vi "Make RomiGyro JSON.vi"(9 "Force":bool, 10 "Previous":T1={"type"="AI", "device"="", "name"="", "data"={"<init"=0, ">connected"=FALSE, "<offsetX"=0.0, "<offsetY"=0.0, "<offsetZ"=0.0, ">angle_x"=0.0, ">angle_y"=0.0, ">angle_z"=0.0, ">rate_x"=0.0, ">rate_y"=0.0, ">rate_z"=0.0, "<gain"=0.0}}, 11 "New":T1={"type"="AI", "device"="", "name"="", "data"={"<init"=0, ">connected"=FALSE, "<offsetX"=0.0, "<offsetY"=0.0, "<offsetZ"=0.0, ">angle_x"=0.0, ">angle_y"=0.0, ">angle_z"=0.0, ">rate_x"=0.0, ">rate_y"=0.0, ">rate_z"=0.0, "<gain"=0.0}}) -> (3 "delta JSON":string)   [LabVIEW 2019]
uses:
  RomiGyro Data proto.ctl
  RomiGyro proto.ctl
panel:
  out "Complete JSON":string
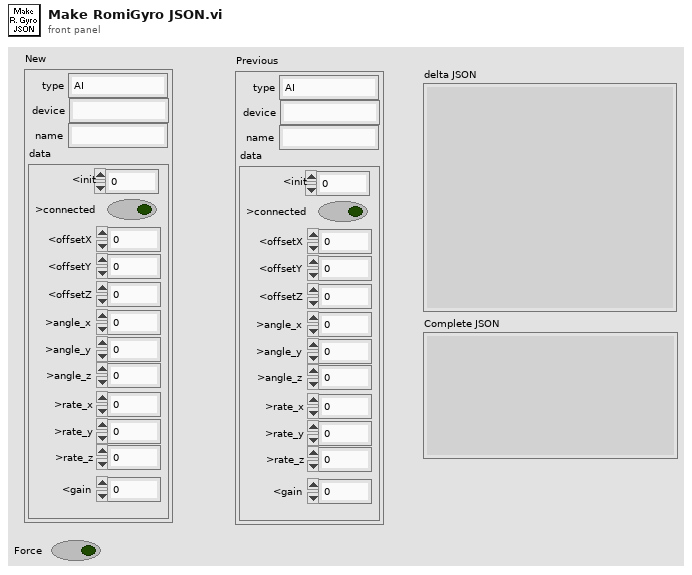
[diagram p1: front panel]
types:
  T1 = typedef "RomiGyro proto.ctl" = cluster{"type":string, "device":string, "name":string, "data":T2}
  T2 = typedef "RomiGyro Data proto.ctl" = cluster{"<init":i32, ">connected":bool, "<offsetX":dbl, "<offsetY":dbl, "<offsetZ":dbl, ">angle_x":dbl, ">angle_y":dbl, ">angle_z":dbl, ">rate_x":dbl, ">rate_y":dbl, ">rate_z":dbl, "<gain":dbl}
  T3 = cluster{"type":bool, "device":bool, "name":bool, "data":cluster{"<init":bool, ">connected":bool, "<offsetX":bool, "<offsetY":bool, "<offsetZ":bool, ">angle_x":bool, ">angle_y":bool, ">angle_z":bool, ">rate_x":bool, ">rate_y":bool, ">rate_z":bool, "<gain":bool}}
  T4 = cluster{"<init":bool, ">connected":bool, "<offsetX":bool, "<offsetY":bool, "<offsetZ":bool, ">angle_x":bool, ">angle_y":bool, ">angle_z":bool, ">rate_x":bool, ">rate_y":bool, ">rate_z":bool, "<gain":bool}
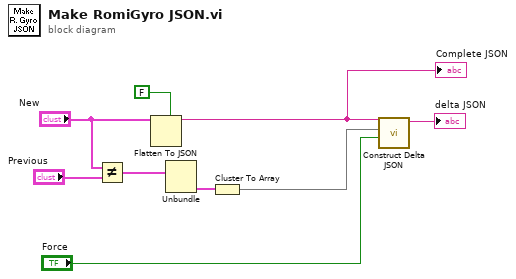
[diagram p0: block diagram]
diagram:
  n1 = Not Equal?(x="New", y="Previous") -> (x != y?=w6:T3)
  n2 = Flatten To JSON(enable LabVIEW extensions? (T)=FALSE, anything="New") -> (JSON string=w5:string)  [unwired: 1 in, 1 out]
  "Complete JSON" <- w5
  n3 = Unbundle(w6) -> ("data"=w2:T4)  [unwired: 3 out]
  n4 = Cluster To Array(cluster=w2) -> (array=w1:bool[])
  n5 = call "Construct Delta JSON.vi"("Force"="Force", "Checked Items"=w1, "JSON string"=w5) -> ("Delta JSON"=→"delta JSON":string)  [unwired: 8 in]
